vi "Build FromVSEngine Command Channels.vi"(8 "error in (no error)":errorcluster, 11 "Injector section ref in":T1 format="%.0x") -> (0 "error out":errorcluster, 1 "WaveformEnable?":T1 format="%.0x", 2 "InjectionSettings":T1[](array[typedef]) format="%.0x", 3 "Injector section ref out":T1 format="%.0x")   [LabVIEW 2019, in "Fuel Injector Analysis Addon System Explorer.lvlib"]
uses:
  Fuel Injector Analysis Addon System Explorer.lvlib
  <vilib>/NI VeriStand/Custom Device API/Custom Device Item Ref.ctl
  Addon Shared/SubVIs/Constants.vi
  <vilib>/NI VeriStand/Custom Device Tools/Custom Device Utility Library/NI VeriStand - Search for Item by GUID.vi
  <vilib>/NI VeriStand/Custom Device Tools/Custom Device Utility Library/NI VeriStand - Search for Item by Name.vi
  <vilib>/NI VeriStand/Custom Device Tools/Custom Device Utility Library/Custom Device Utility Library.lvlib
  Addon Shared/Fuel Injector Analysis Addon Shared.lvlib
  <vilib>/NI VeriStand/Custom Device API/Custom Device API.lvlib
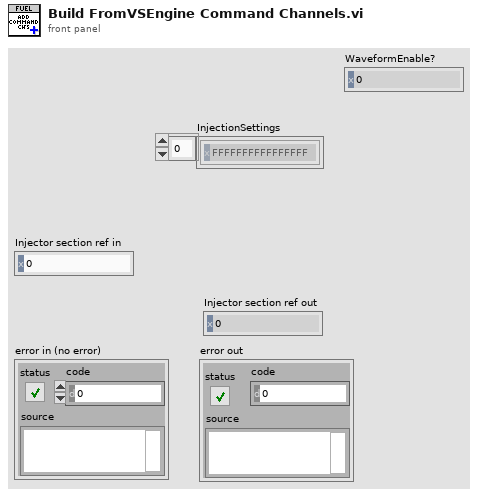
[diagram p1: front panel]
types:
  T1 = typedef "Custom Device API.lvlib/Custom Device Item Ref.ctl" = u64
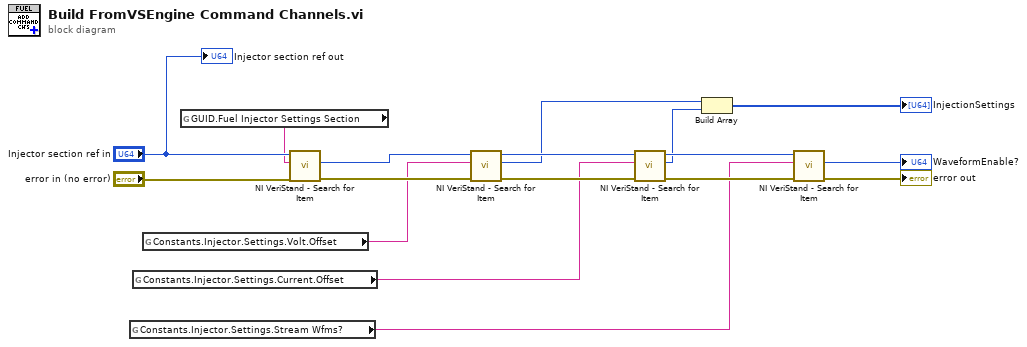
[diagram p0: block diagram]
diagram:
  n1 = global read "Constants.vi" "Constants.Injector.Settings.Stream Wfms?"() -> (w7:string)
  n2 = global read "Constants.vi" "Constants.Injector.Settings.Current.Offset"() -> (w6:string)
  n3 = global read "Constants.vi" "Constants.Injector.Settings.Volt.Offset"() -> (w5:string)
  n4 = global read "Constants.vi" "GUID.Fuel Injector Settings Section"() -> (w15:string)
  n5 = call-poly <vilib>:"NI VeriStand - Search for Item.vi"("error in"="error in (no error)", "Item GUID"=w15, "Section Ref in"="Injector section ref in") -> ("error out"=w14:errorcluster, "Item Ref"=w13:T1)  [unwired: 5 in, 2 out]
  n6 = call-poly <vilib>:"NI VeriStand - Search for Item.vi"("error in"=w14, "Item Name"=w5, "Section Ref in"=w13) -> ("error out"=w12:errorcluster, "Item Ref"=w3:T1, "Section Ref out"=w9:T1)  [unwired: 5 in, 1 out]
  n7 = call-poly <vilib>:"NI VeriStand - Search for Item.vi"("error in"=w12, "Item Name"=w6, "Section Ref in"=w9) -> ("error out"=w11:errorcluster, "Item Ref"=w2:T1, "Section Ref out"=w8:T1)  [unwired: 5 in, 1 out]
  n8 = Build Array(w3, w2) -> (→"InjectionSettings":T1[])
  n9 = call-poly <vilib>:"NI VeriStand - Search for Item.vi"("error in"=w11, "Item Name"=w7, "Section Ref in"=w8) -> ("error out"=→"error out":errorcluster, "Item Ref"=→"WaveformEnable?":T1)  [unwired: 5 in, 2 out]
  "Injector section ref out" <- "Injector section ref in"
